vi "PCI Configuration Vendor ID.Get.vi"(8 "error in (no error)":errorcluster, 11 "GE 5565PIORC":refnum<class "GE 5565PIORC.lvclass">) -> (0 "error out":errorcluster, 2 "Vendor ID":u16, 3 "GE 5565PIORC out":refnum<class "GE 5565PIORC.lvclass">)   [LabVIEW 2016, in "GE 5565PIORC.lvclass"]
uses:
  GE 5565PIORC.lvclass
  <vilib>/Instr/_visa.llb/VISA Register Access Address Space.ctl
  Controls/Registers.PCI Configuration.ctl
  GE 5565PIORC.lvclass/GE 5565PIORC.ctl
  Binary Operations/Get Bits U32.vi
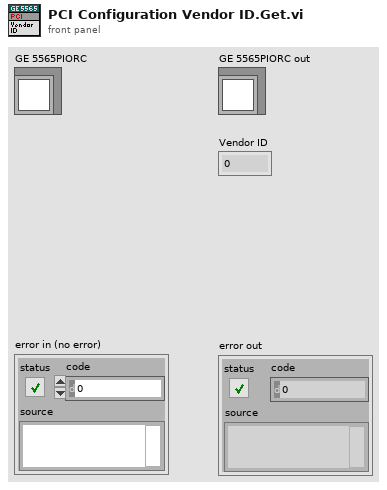
[diagram p1: front panel]
types:
  T1 = typedef "GE 5565PIORC.lvclass/Registers.PCI Configuration.ctl" = enum16{"PCI Configuration ID", "PCI Command", "PCI Status", "PCI Revision ID", "PCI Class Code", "PCI Cache Line Size", "PCI Latency Timer", "PCI Header Type", "PCI Built-In Self-Test", "PCI BAR 0", "PCI BAR 1", "PCI BAR 2", "PCI BAR 3", "PCI BAR 4", "PCI BAR 5", "PCI Cardbus CIS Pointer", "PCI Subsystem Vendor ID", "PCI Subsytem ID", "PCI Expansion ROM Base", "PCI Capability Pointer", "PCI Interrupt Line", "PCI Interrupt Pin", "PCI Min_Gnt", "PCI Max_Lat"}
  T2 = typedef "VISA Register Access Address Space.ctl" = u16
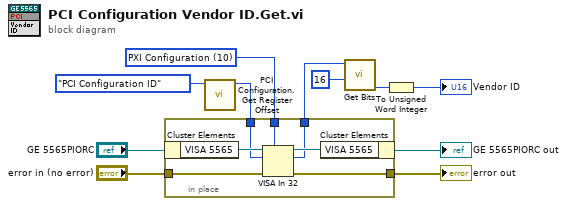
[diagram p0: block diagram]
diagram:
  w4 = T2 10 items=["VXI/VME A16"=1, "VXI/VME A24"=2, "VXI/VME A32"=3, "VXI/VME A64"=4, "PXI Memory Allocations"=9, "PXI Configuration"=10, "PXI BAR0"=11, "PXI BAR1"=12, "PXI BAR2"=13, "PXI BAR3"=14, "PXI BAR4"=15, "PXI BAR5"=16] ("Address Space")
  n1 = call "PCI Configuration.Get Register Offset.vi"("PCI Configuration Register"=Registers.PCI_Configuration."PCI Configuration ID") -> ("Offset"=w1:u32)  [unwired: 10 in]
  n2 = in-place {
    in-place-border: "error in (no error)" -> [w16]
    in-place-border: [w15] -> w6
    in-place-border: w1 -> [w14]
    in-place-border: w4 -> [w13]
    in-place-border: [w12] -> w3
    n3 = in-place-cluster #1("GE 5565PIORC") -> ("VISA 5565"=w18:refnum<visa-resource-name>)
    n4 = VISA In 32(7:w13, 8:w16, 10:w14, 11:w18) -> (0:w15:errorcluster, 2:w12:u32, 3:w17:refnum<visa-resource-name>)
    n5 = in-place-cluster #1("VISA 5565"=w17) -> (→"GE 5565PIORC out":refnum<class "GE 5565PIORC.lvclass">)
  }
  "error out" <- w6
  n6 = call-poly "Get Bits.vi"("Length (1)"=u8 16, "Register in"=w3) -> ("Value"=w11:u32)  [unwired: 6 in, 3 out]
  n7 = To Unsigned Word Integer(number=w11) -> (unsigned 16bit integer=→"Vendor ID":u16)
